vi "Init.vi"(8 "error in (no error)":errorcluster, 10 "url (\"/mcp/server\")":string="/mcp/server", 11 "id":i32) -> (0 "error out":errorcluster, 3 "MCP Handler out":refnum<class "MCP Handler.lvclass">)   [LabVIEW 2020, in "MCP Server.lvlib" / "MCP Handler.lvclass"]
uses:
  MCP Handler.lvclass
  MCP Handler.lvclass/MCP Handler.ctl
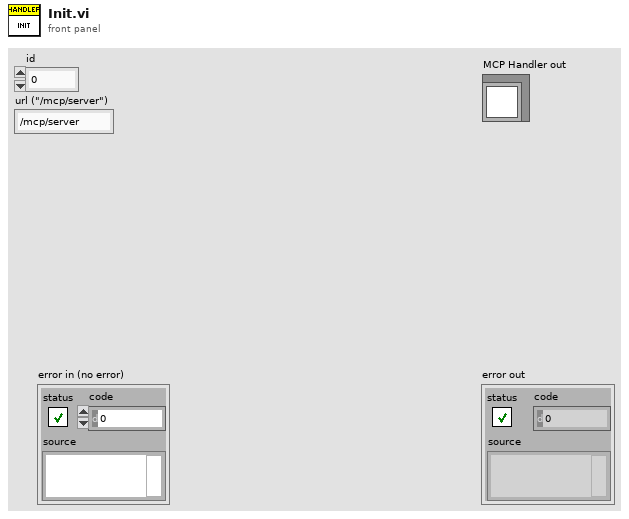
[diagram p1: front panel]
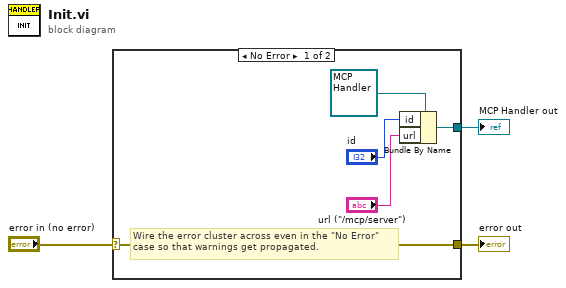
[diagram p0: block diagram]
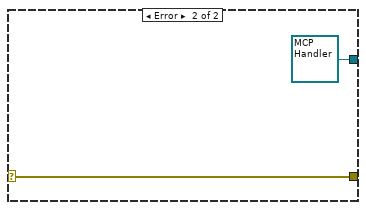
[diagram p2: hidden frame]
diagram:
  n1 = case shown="No Error" "error in (no error)" {
    selector: "error in (no error)" -> [w8 w10]
    tunnel: [w8 w10] -> w2
    tunnel: [w6 refnum<class "MCP Handler.lvclass"> refnum ("MCP Handler in")] -> w1
    frame No Error {
      # "Wire the error cluster across even in the \"No Error\"\ncase so that warnings get propagated."
      n2 = Bundle By Name(cluster=refnum<class "MCP Handler.lvclass"> refnum ("MCP Handler in"), "id"="id", "url"="url (\"/mcp/server\")") -> (w6:refnum<class "MCP Handler.lvclass">)
    }
    frame Error {
    }
  }
  "error out" <- w2
  "MCP Handler out" <- w1
